vi "get ring string.vi"(10 "error in":errorcluster, 11 "Ring in":refnum<vi>) -> (2 "error out":errorcluster, 3 "String":string)   [LabVIEW 2013, in "fixed channel tag bus module editor node.lvclass"]
uses:
  fixed channel tag bus module editor node.lvclass
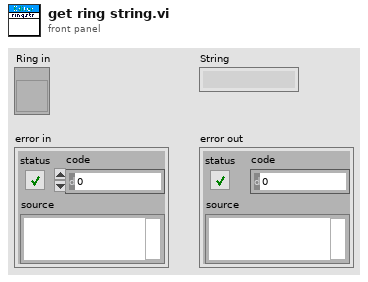
[diagram p1: front panel]
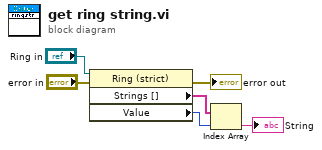
[diagram p0: block diagram]
diagram:
  n1 = property on="Property Node" class="Ring (strict)"(reference="Ring in", error in="error in") -> (error out=→"error out":errorcluster, "Strings []"=w3:string[], "Value"=w6:u16)  [unwired: 1 out]
  n2 = Index Array(array=w3, index=w6) -> (element=→"String":string)
